vi "Rotate Z-axis.vi"(6 "angle unit":u16(ring) items=["degree", "radians"], 7 "Relative?":bool, 8 "error in (no error)":errorcluster, 10 "angle":sgl, 11 "Scene Object In":refnum<vi>) -> (0 "error out":errorcluster, 3 "Scene Object Out":refnum<vi>)   [LabVIEW 2020, in "NI_3D Picture Control.lvlib"]
doc: "Rotates an object about the Z-axis."
uses:
  <vilib>/picture/3D Picture Control/NI_3D Picture Control.lvlib
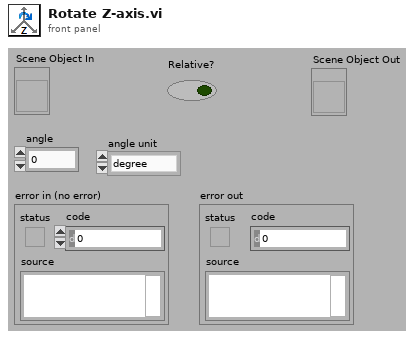
[diagram p1: front panel]
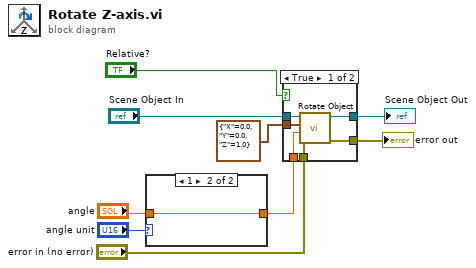
[diagram p0: block diagram]
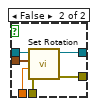
[diagram p2: hidden frame]
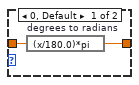
[diagram p3: hidden frame]
diagram:
  n1 = case shown="1" "angle unit" {
    tunnel: "angle" -> [w11 w12]
    tunnel: [w10 w12] -> w4
    frame 0, Default {
      n2 = expression code="(x/180.0)*pi" "degrees to radians"(w11) -> (w10:sgl)
    }
    frame 1 {
    }
  }
  n3 = case shown="True" "Relative?" {
    tunnel: "error in (no error)" -> [w18 w24]
    tunnel: "Scene Object In" -> [w17 w23]
    tunnel: [w16 w22] -> w7
    tunnel: [w15 w21] -> w6
    tunnel: w4 -> [w14 w20]
    tunnel: cluster{"X":sgl, "Y":sgl, "Z":sgl} {"X"=0.0, "Y"=0.0, "Z"=1.0} ("Axis") -> [w13 w19]
    frame True {
      n4 = call <vilib>:"Rotate Object.vi"("error in (no error)"=w18, "Angle"=w14, "Axis"=w13, "Scene.Object In"=w17) -> ("error out"=w15:errorcluster, "Scene.Object Out"=w16:refnum<vi>)  [unwired: 6 in]
    }
    frame False {
      n5 = call <vilib>:"Set Rotation.vi"("error in (no error)"=w24, "Angle"=w20, "Axis"=w19, "Scene Object"=w23) -> ("error out"=w21:errorcluster, "Rotated Scene Object"=w22:refnum<vi>)  [unwired: 6 in]
    }
  }
  "Scene Object Out" <- w7
  "error out" <- w6
